vi "NI-DAQ Synthesizer.vi"(5 "Start counter":bool, 6 "Resources to use":T1={"Counter"="ctr0", "Analog Out"="ao0", "Counter output terminal"=" "}, 7 "Amplitude, V":dbl=1.0 format="%0.2f", 8 "error in":errorcluster, 9 "Samples per sine wave":i32=100, 10 "Sine frequency, Hz":dbl=1000.0 format="%#_6p", 11 "DAQmx Device Name":tag) -> (0 "error out":errorcluster, 1 "DAQ Clock channel name":string, 2 "AO task out":refnum<k21>, 3 "Counter task out":refnum<k21>)   [LabVIEW 2020]
uses:
  <vilib>/DAQmx/write.llb/DAQmx Write (Analog 1D DBL 1Chan NSamp).vi
  <vilib>/DAQmx/create/channels.llb/DAQmx Create Channel (CO-Pulse Generation-Frequency).vi
  <vilib>/DAQmx/configure/timing.llb/DAQmx Timing (Implicit).vi
  <vilib>/DAQmx/create/channels.llb/DAQmx Create Channel (AO-Voltage-Basic).vi
  <vilib>/DAQmx/configure/timing.llb/DAQmx Timing (Sample Clock).vi
  <vilib>/DAQmx/miscellaneous.llb/DAQmx Fill In Error Info.vi
  <vilib>/Analysis/NI_AALPro.lvlib
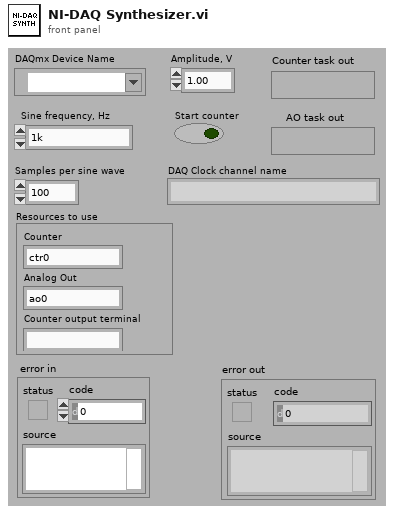
[diagram p1: front panel]
types:
  T1 = cluster{"Counter":string, "Analog Out":string, "Counter output terminal":string}
  T2 = enum16{"sine", "cosine", "triangle", "square", "sawtooth", "increasing ramp", "decreasing ramp"}
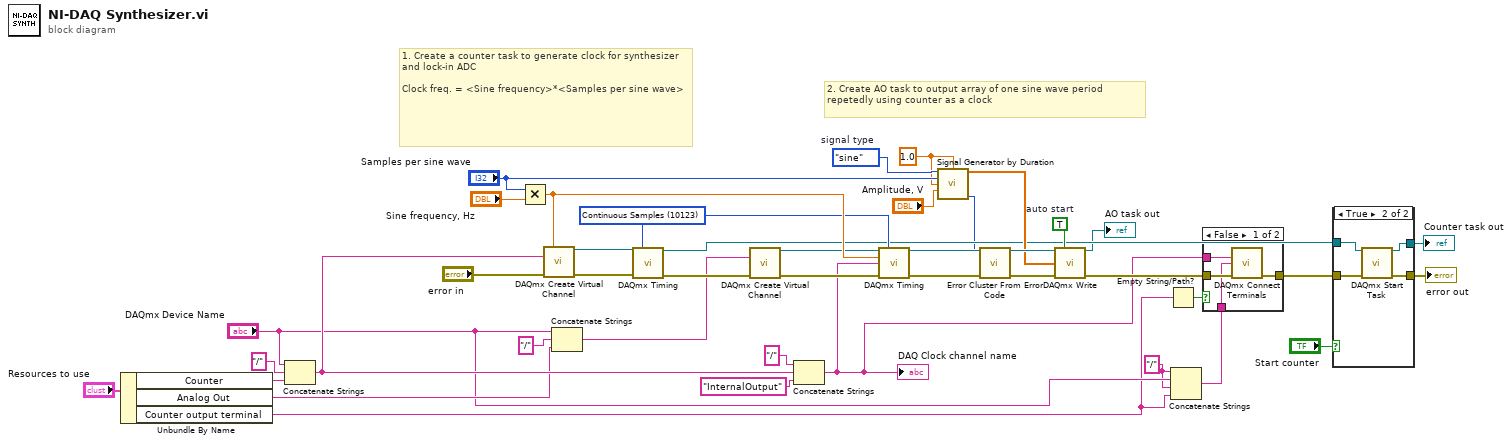
[diagram p0: block diagram]
diagram:
  w1 = "/"
  w20 = 1.0 ("duration")
  w37 = TRUE  # auto start
  w33 = T2."sine"  # signal type
  w24 = 10123 items=["Finite Samples"=10178, "Continuous Samples"=10123, "Hardware Timed Single Point"=12522] ("sample mode")
  # "2. Create AO task to output array of one sine wave period repetedly using counter as a clock"
  # "1. Create a counter task to generate clock for synthesizer and lock-in ADC \n\nClock freq. = <Sine frequency>*<Samples per sine wave>"
  n1 = Unbundle By Name("Resources to use") -> ("Counter"=w17:string, "Analog Out"=w16:string, "Counter output terminal"=w3:string)
  n2 = Concatenate Strings("DAQmx Device Name", "/", w17) -> (w32:string)
  n3 = Multiply(x="Samples per sine wave", y="Sine frequency, Hz") -> (x*y=w41:dbl)
  n4 = call-poly <vilib>:"DAQmx Create Virtual Channel.vi"("frequency"=w41, "counter"=w32, "error in"="error in") -> ("task out"=w29:refnum<k21>, "error out"=w21:errorcluster)  [unwired: 6 in, 5 out]
  n5 = Concatenate Strings("DAQmx Device Name", "/", w16) -> (w26:string)
  n6 = call-poly <vilib>:"DAQmx Timing.vi"("task/channels in"=w29, "sample mode"=w24, "error in"=w21) -> ("task out"=w23:refnum<k21>, "error out"=w38:errorcluster)  [unwired: 11 in]
  n7 = call-poly <vilib>:"DAQmx Create Virtual Channel.vi"("physical channels"=w26, "error in"=w38) -> ("task out"=w27:refnum<k21>, "error out"=w12:errorcluster)  [unwired: 7 in, 5 out]
  n8 = Concatenate Strings("/", w32, "InternalOutput" ("string")) -> (w5:string)
  "DAQ Clock channel name" <- w5
  n9 = call-poly <vilib>:"DAQmx Timing.vi"("task/channels in"=w27, "sample mode"=w24, "rate"=w41, "source"=w5, "error in"=w12) -> ("task out"=w36:refnum<k21>, "error out"=w11:errorcluster)  [unwired: 2 in, 7 out]
  n10 = call <vilib>:"Signal Generator by Duration.vi"("signal type"=w33, "duration"=w20, "# of samples"="Samples per sine wave", "frequency"=w20, "amplitude"="Amplitude, V") -> ("signal"=w35:dbl[], "error"=w22:i32)  [unwired: 7 in, 2 out]
  n11 = call <vilib>:"Error Cluster From Error Code.vi"("error in (no error)"=w11, "error code (0)"=w22) -> ("error out"=w10:errorcluster)  [unwired: 7 in]
  n12 = call-poly <vilib>:"DAQmx Write.vi"("task/channels in"=w36, "auto start"=w37, "data"=w35, "error in"=w10) -> ("task out"=→"AO task out":refnum<k21>, "error out"=w8:errorcluster)  [unwired: 10 out]
  n13 = Empty String/Path?(string/path=w3) -> (empty?=w6:bool)
  n14 = Concatenate Strings(w1, "DAQmx Device Name", w1, w3) -> (w2:string)
  n15 = case shown="False" w6 {
    tunnel: w8 -> [w45 w46]
    tunnel: [w44 w46] -> w7
    tunnel: w5 -> [w43 _]
    tunnel: w2 -> [w42 _]
    frame False {
      n16 = call <vilib>:"DAQmx Connect Terminals.vi"("source terminal"=w43, "destination terminal"=w42, "error in"=w45) -> ("error out"=w44:errorcluster)  [unwired: 12 in]
    }
    frame True {
    }
  }
  n17 = case shown="True" "Start counter" {
    tunnel: w23 -> [w48 w52]
    tunnel: w7 -> [w47 w51]
    tunnel: [w47 w50] -> w19
    tunnel: [w48 w49] -> w13
    frame False {
    }
    frame True {
      n18 = call <vilib>:"DAQmx Start Task.vi"("task/channels in"=w52, "error in"=w51) -> ("task out"=w49:refnum<k21>, "error out"=w50:errorcluster)  [unwired: 12 in]
    }
  }
  "error out" <- w19
  "Counter task out" <- w13
